vi "checksum.vi"() -> ()   [LabVIEW 2019]
panel:
  in  "array 2":u8[](array[numeric])
  out "Sum":u32
  out "Check sum":u16
  in  "array":u8[](array[numeric])
  out "Data":u16
  in  "Index":i32
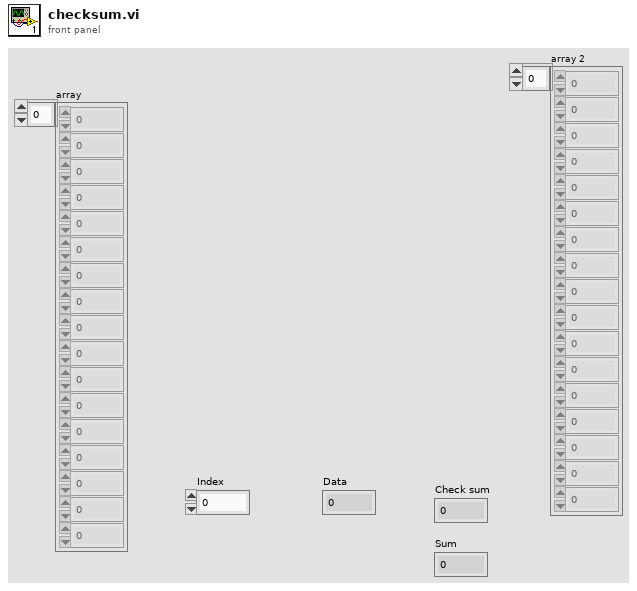
[diagram p1: front panel]
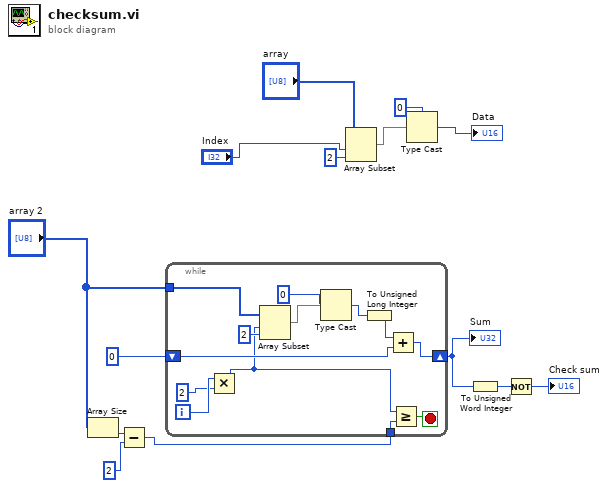
[diagram p0: block diagram]
diagram:
  n1 = Array Size(array="array 2") -> (size(s)=w7:i32)
  n2 = Subtract(x=w7, y=2) -> (x-y=w6:i32)
  n3 = while {
    tunnel: "array 2" -> [w16]
    shift-right: [w24] -> w5
    shift-left: u32 0 ("(hi.lo)") -> [w25]
    tunnel: w6 -> [w22]
    i -> [w27]
    stop <- w23 stop-if-true
    n4 = Multiply(x=w27, y=2) -> (x*y=w15:i32)
    n5 = Array Subset(array=w16, index=w15, length=2) -> (w21:u8[])
    n6 = Type Cast(type=u16 0 ("Data"), x=w21) -> (*(type *) &x=w19:u16)
    n7 = To Unsigned Long Integer(number=w19) -> (unsigned 32bit integer=w17:u32)
    n8 = Add(x=w17, y=w25) -> (x+y=w24:u32)
    n9 = Greater Or Equal?(x=w15, y=w22) -> (x >= y?=w23:bool)
  }
  "Sum" <- w5
  n10 = Array Subset(array="array", index="Index", length=2) -> (w12:u8[])
  n11 = Type Cast(type=u16 0 ("Data"), x=w12) -> (*(type *) &x=→"Data":u16)
  n12 = To Unsigned Word Integer(number=w5) -> (unsigned 16bit integer=w4:u16)
  n13 = Not(x=w4) -> (.not. x?=→"Check sum":u16)
